vi "Get Instrument Paths.vi"() -> (0 "paths":path[](array[path]))   [LabVIEW 2021]
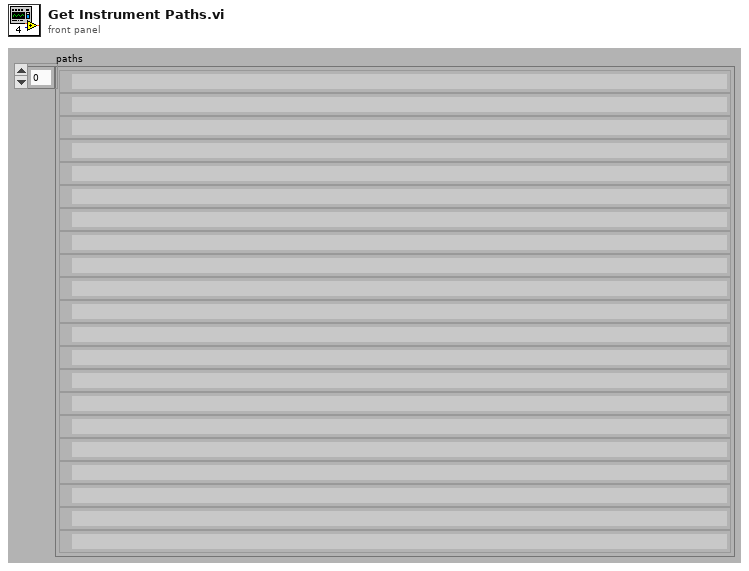
[diagram p1: front panel]
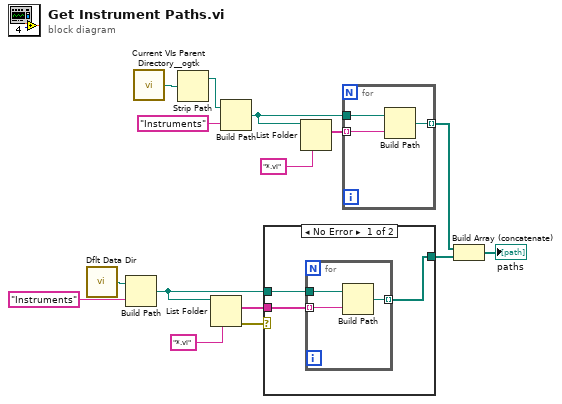
[diagram p0: block diagram]
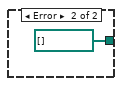
[diagram p2: hidden frame]
diagram:
  n1 = call <vilib>:"Dflt Data Dir.vi"() -> ("App:Default Data Directory"=w8:path)
  n2 = Build Path(base path=w8, name or relative path="Instruments") -> (appended path=w3:path)
  n3 = call <userlib>:"Current VIs Parent Directory__ogtk.vi"() -> ("Parent Directory (+ Relative)"=w10:path)  [unwired: 5 in]
  n4 = Strip Path(path=w10) -> (stripped path=w11:path)  [unwired: 1 out]
  n5 = List Folder(path=w3, pattern="*.vi") -> (filenames=w4:string[], error out=w1:errorcluster)  [unwired: 2 in, 2 out]
  n6 = Build Path(base path=w11, name or relative path="Instruments") -> (appended path=w13:path)
  n7 = case shown="No Error" w1 {
    tunnel: w4 -> [w18 _]
    tunnel: w3 -> [w17 _]
    tunnel: [w16 path[] []] -> w2
    frame No Error {
      n8 = for {
        tunnel: [w21] -> w16 mode=indexing
        tunnel: w17 -> [w20]
        tunnel: w18 -> [w19] mode=indexing
        n9 = Build Path(base path=w20, name or relative path=w19) -> (appended path=w21:path)
      }
    }
    frame Error {
    }
  }
  n10 = List Folder(path=w13, pattern="*.vi") -> (filenames=w12:string[])  [unwired: 2 in, 3 out]
  n11 = for {
    tunnel: [w25] -> w5 mode=indexing
    tunnel: w13 -> [w24]
    tunnel: w12 -> [w23] mode=indexing
    n12 = Build Path(base path=w24, name or relative path=w23) -> (appended path=w25:path)
  }
  n13 = Build Array (concatenate)(w5, w2) -> (→"paths":path[])
